vi "Close.vi"(8 "error in (no error)":errorcluster, 11 "Sink-Console in":refnum<class "Sink-Console.lvclass">) -> (0 "error out":errorcluster, 3 "Sink-Console out":refnum<class "Sink-Console.lvclass">)   [LabVIEW 2019, in "TSC Event Logger.lvlib" / "Sink-Console.lvclass"]
uses:
  Sink-Console.lvclass
  Sink-Console.lvclass/Sink-Console.ctl
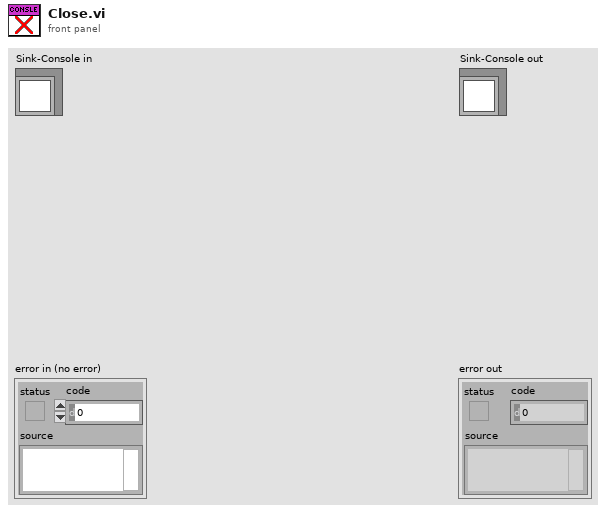
[diagram p1: front panel]
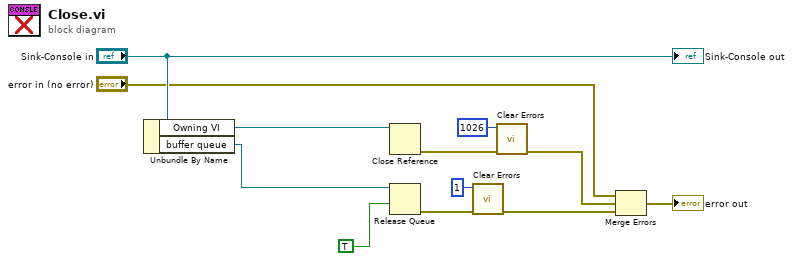
[diagram p0: block diagram]
diagram:
  n1 = Unbundle By Name("Sink-Console in") -> ("Owning VI"=w7:refnum<vi>, "buffer queue"=w10:refnum<queue>)
  n2 = Close Reference(reference=w7) -> (error out=w6:errorcluster)  [unwired: 1 in]
  n3 = Release Queue(queue=w10, force destroy? (F)=TRUE) -> (error out=w11:errorcluster)  [unwired: 1 in, 2 out]
  n4 = call <vilib>:"Clear Errors.vi"("error in (no error)"=w11, "specific error code to clear (0: all)"=1) -> ("error out"=w2:errorcluster)  [unwired: 4 in, 1 out]
  n5 = call <vilib>:"Clear Errors.vi"("error in (no error)"=w6, "specific error code to clear (0: all)"=1026) -> ("error out"=w5:errorcluster)  [unwired: 4 in, 1 out]
  n6 = Merge Errors("error in (no error)", w5, w2) -> (→"error out":errorcluster)
  "Sink-Console out" <- "Sink-Console in"
